vi "create received data message.vi"(11 "data":refnum<class "communicator message.lvclass">) -> (3 "message":refnum<class "communicator message.lvclass">)   [LabVIEW 2015, in "queue manager.lvclass"]
uses:
  queue manager.lvclass
  message/communicator message.lvclass
  message/communicator message.lvclass/communicator message.ctl
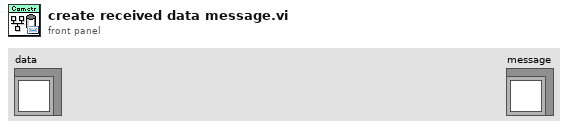
[diagram p1: front panel]
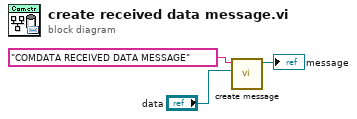
[diagram p0: block diagram]
diagram:
  n1 = call "create message.vi"("data"="data", "ID"="COMDATA RECEIVED DATA MESSAGE") -> ("message"=→"message":refnum<class "communicator message.lvclass">)  [unwired: 9 in]
